vi "beepMulti.vi"(10 "Time":i32) -> ()   [LabVIEW 2010]
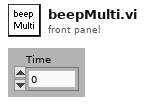
[diagram p1: front panel]
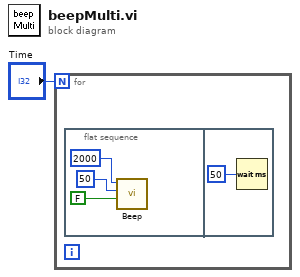
[diagram p0: block diagram]
diagram:
  n1 = for {
    N: "Time" -> [_]
    n2 = flat-sequence {
      frame #0 {
        n3 = call <vilib>:"Beep.vi"("use system alert? (T)"=FALSE, "duration (msec)"=u32 50, "frequency (Hz)"=u32 2000) -> ()  [unwired: 9 in]
      }
      frame #1 {
        n4 = Wait (ms)(milliseconds to wait=u32 50 ("等待时间（毫秒）")) -> ()  [unwired: 1 out]
      }
    }
  }
